vi "Optomize Settings.vi"(5 "Aviod Zone":cluster{"pos 1":dbl, "pos 2":dbl} {"pos 1" format="%#.3g"; "pos 2" format="%#.3g"}, 7 "Previous Swerve Setting":T1 {"Back Right"."Angle" scale format="%.3f"; "Back Right"."Velocity" scale=-1.0..1.0 scale format="%.1f"; "Back Left"."Angle" scale format="%.3f"; "Back Left"."Velocity" scale=-1.0..1.0 scale format="%.1f"; "Front Left"."Angle" scale format="%.3f"; "Front Left"."Velocity" scale=-1.0..1.0 scale format="%.1f"; "Front Right"."Angle" scale format="%.3f"; "Front Right"."Velocity" scale=-1.0..1.0 scale format="%.1f"}, 11 "Swerve Request":T1 {"Back Right"."Angle" scale format="%.3f"; "Back Right"."Velocity" scale=-1.0..1.0 scale format="%.1f"; "Back Left"."Angle" scale format="%.3f"; "Back Left"."Velocity" scale=-1.0..1.0 scale format="%.1f"; "Front Left"."Angle" scale format="%.3f"; "Front Left"."Velocity" scale=-1.0..1.0 scale format="%.1f"; "Front Right"."Angle" scale format="%.3f"; "Front Right"."Velocity" scale=-1.0..1.0 scale format="%.1f"}) -> (3 "Swerve Setting Out":T1 {"Back Right"."Angle" scale format="%.3f"; "Back Right"."Velocity" scale=-1.0..1.0 scale format="%.1f"; "Back Left"."Angle" scale format="%.3f"; "Back Left"."Velocity" scale=-1.0..1.0 scale format="%.1f"; "Front Left"."Angle" scale format="%.3f"; "Front Left"."Velocity" scale=-1.0..1.0 scale format="%.1f"; "Front Right"."Angle" scale format="%.3f"; "Front Right"."Velocity" scale=-1.0..1.0 scale format="%.1f"})   [LabVIEW 2023, in "TShirtWork-SwerveDrive_ACT_ts.lvlib"]
uses:
  TShirtWork-SwerveDrive_ACT_ts.lvlib
  Shared Code/TypeDefs/Level_Velocity plus-minus 1.ctl
  Shared Code/TypeDefs/Dial_Compase heading unit circle CCW positive.ctl
  Shared Code/TypeDefs/Cluster_Module Velocity-Direction-Rotations.ctl
  Shared Code/TypeDefs/Cluster_Swerve 4 Steer and Velocity.ctl
panel:
  # "\"Front\" of Robot"
  # "Right Hand Rule"
  # "X"
  # "+CCW"
  # "Y"
  # "(0,0)"
  # "\"Front\" of Robot"
  # "Right Hand Rule"
  # "X"
  # "+CCW"
  # "Y"
  # "(0,0)"
  # "\"Front\" of Robot"
  # "Right Hand Rule"
  # "X"
  # "+CCW"
  # "Y"
  # "(0,0)"
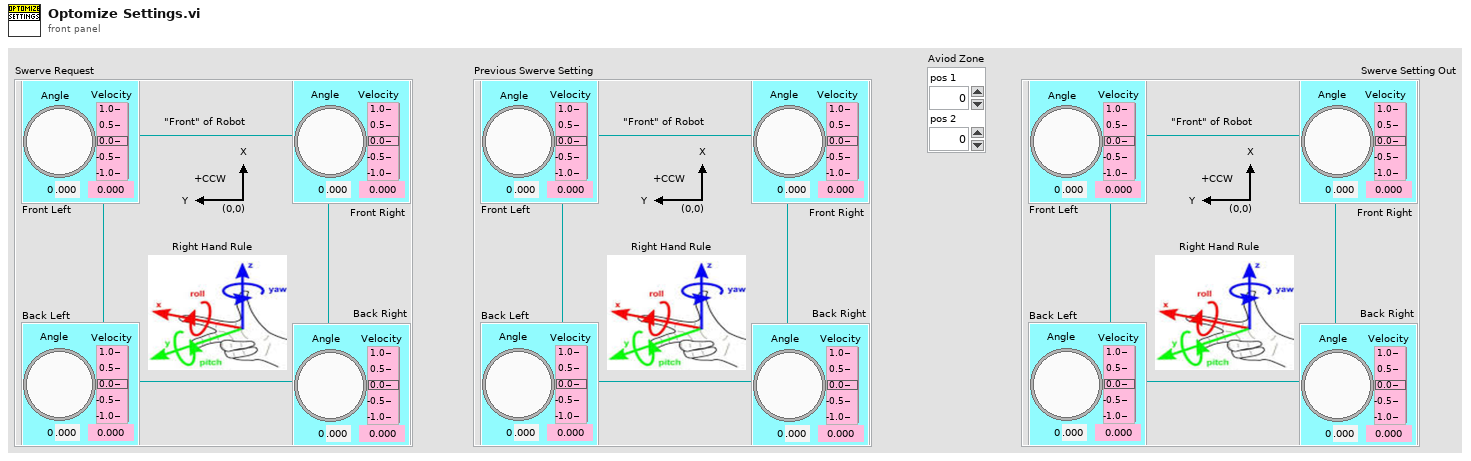
[diagram p1: front panel]
types:
  T1 = typedef "Cluster_Swerve 4 Steer and Velocity.ctl" = cluster{"Front Right":T2, "Front Left":T2, "Back Left":T2, "Back Right":T2}
  T2 = typedef "Cluster_Module Velocity-Direction-Rotations.ctl" = cluster{"Velocity":T3, "Angle":T4, "Rotations Count":dbl}
  T3 = typedef "Level_Velocity plus-minus 1.ctl" = dbl
  T4 = typedef "Dial_Compase heading unit circle CCW positive.ctl" = dbl
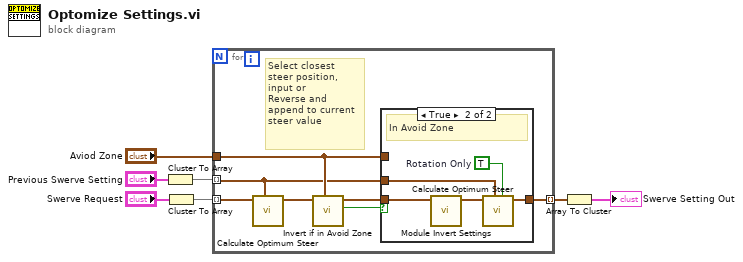
[diagram p0: block diagram]
diagram:
  n1 = Cluster To Array(cluster="Previous Swerve Setting") -> (array=w3:T2[])
  n2 = Cluster To Array(cluster="Swerve Request") -> (array=w5:T2[])
  n3 = for {
    tunnel: w5 -> [w9] mode=indexing
    tunnel: "Aviod Zone" -> [w12]
    tunnel: w3 -> [w11] mode=indexing
    tunnel: [w10] -> w2 mode=indexing
    # "Select closest\nsteer position,\ninput or\nReverse and\nappend to current\nsteer value"
    n4 = call "Calculate Optimum Steer.vi"("Previous Set Swerve"=w11, "New Swerve"=w9) -> ("Set Swerve Out"=w14:T2)  [unwired: 9 in]
    n5 = call "Invert if in Avoid Zone.vi"("Avoid Zone (Unit Circle)"=w12, "Set Values"=w14) -> ("In Avoid Zone"=w13:bool, "Set Values Out"=w8:T2)  [unwired: 8 in]
    n6 = case shown="True" w13 {
      tunnel: w12 -> [_ _]
      tunnel: w11 -> [_ w20]
      tunnel: [w15 w19] -> w10
      tunnel: w8 -> [w15 w17]
      frame False {
        # "Not in Avoid Zone"
      }
      frame True {
        w16 = TRUE  # Rotation Only
        # "In Avoid Zone"
        n7 = call "Module Invert Settings.vi"("Setting"=w17) -> ("Inverted Setting Out"=w18:T2)  [unwired: 10 in]
        n8 = call "Calculate Optimum Steer.vi"("Rotation Only"=w16, "Previous Set Swerve"=w20, "New Swerve"=w18) -> ("Set Swerve Out"=w19:T2)  [unwired: 8 in]
      }
    }
  }
  n9 = Array To Cluster(array=w2) -> (cluster=→"Swerve Setting Out":cluster{"[0]":T2, "[1]":T2, "[2]":T2, "[3]":T2})
